vi "arm driver control.vi"(1 "Joystick Y":dbl) -> (0 "Setpoint":dbl)   [LabVIEW 2014]
uses:
  global variables/devrefs.vi
panel:
  # "Control the arm with PID setpoints instead of direct motor control"
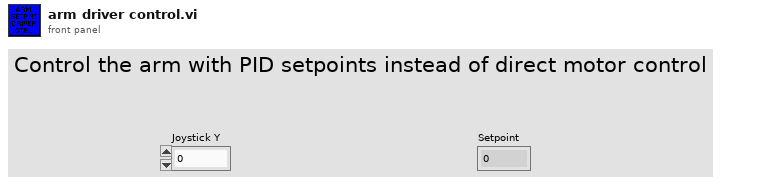
[diagram p1: front panel]
types:
  T1 = typedef "WPI_EncoderDevRef.ctl" = cluster{"DevStatus":errorcluster, "EncoderIndex":T2, "CounterIndex":T3, "DistancePerCount":dbl, "Decoding Type":T4}
  T2 = typedef "FPGA_EncoderIdx.ctl" = enum8{"Enc 0", "Enc 1", "Enc 2", "Enc 3", "Enc 4", "Enc 5", "Enc 6", "Enc 7", "Invalid"}
  T3 = typedef "FPGA_CounterCtrSystemIndex.ctl" = enum8{"Ctr 0", "Ctr 1", "Ctr 2", "Ctr 3", "Ctr 4", "Ctr 5", "Ctr 6", "Ctr 7", "Invalid"}
  T4 = typedef "WPI_EncoderType.ctl" = enum16{"1x", "2x", "4x"}
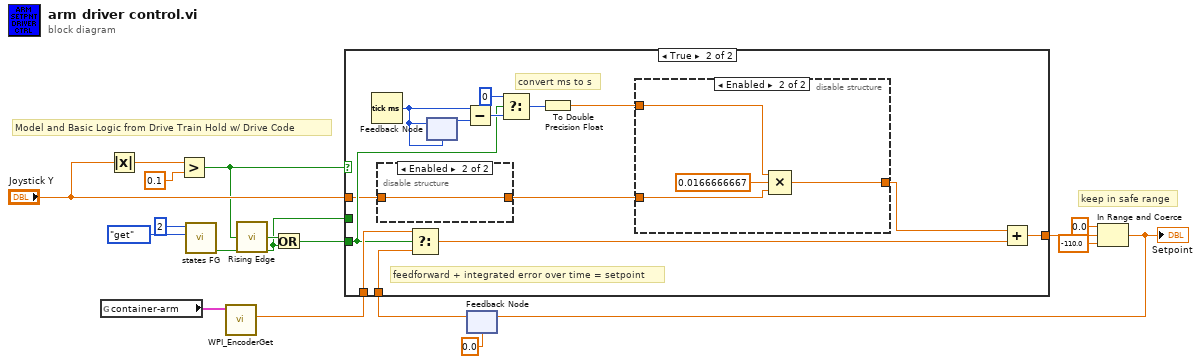
[diagram p0: block diagram]
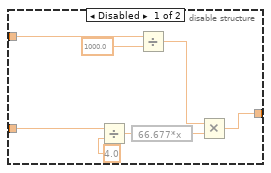
[diagram p4: hidden frame]
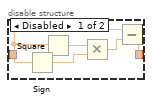
[diagram p5: hidden frame]
diagram:
  # "keep in safe range"
  # "Model and Basic Logic from Drive Train Hold w/ Drive Code"
  n1 = global read "devrefs.vi" "container-arm"() -> (w5:T1)
  n2 = Absolute Value(x="Joystick Y") -> (abs(x)=w16:dbl)
  n3 = Greater?(x=w16, y=0.1) -> (0:w10:bool)
  n4 = call "states FG.vi"("menu (get)"=enum16{"set", "get"}."get", "Loop ID"=2) -> ("first call?"=w6:bool)  [unwired: 6 in, 3 out]
  n5 = call <vilib>:"WPI_EncoderGet.vi"("EncoderDevRef"=w5) -> ("Distance"=w9:dbl)  [unwired: 5 in, 5 out]
  n6 = call "Rising Edge.vi"("Input"=w10) -> ("Rising Edge"=w12:bool)
  n7 = Or(x=w12, y=w6) -> (x .or. y?=w7:bool)
  n8 = feedback #1(0.0 ("upper limit")) -> (w8:dbl)
  n9 = case shown="True" w10 {
    tunnel: "Joystick Y" -> [_ w30]
    tunnel: w8 -> [w21 w35]
    tunnel: w7 -> [_ w31]
    tunnel: w9 -> [w20 w34]
    tunnel: [w19 w28] -> w4
    tunnel: w6 -> [w18 _]
    frame False {
      n10 = case shown="True" w18 {
        tunnel: w21 -> [w22 _]
        tunnel: w20 -> [_ w23]
        tunnel: [w22 w23] -> w19
        frame False {
          # "and get it there if it isn't there"
          # "hold arm at current commanded location"
        }
        frame True {
          # "hold arm at encoder location"
        }
      }
    }
    frame True {
      # "feedforward + integrated error over time = setpoint"
      # "convert ms to s"
      n11 = Tick Count (ms)() -> (millisecond timer value=w25:u32)
      n12 = disable-structure shown="Enabled" {
        disable-tunnel: w30 -> [w54 w55]
        disable-tunnel: [w53 w55] -> w27
        frame Disabled {
          n13 = Sign(1:w54) -> (0:w51:dbl)
          n14 = Square(x=w54) -> (x^2=w52:dbl)
          n15 = Multiply(x=w52, y=w51) -> (x*y=w50:dbl)
          n16 = Subtract(x=w54, y=w50) -> (x-y=w53:dbl)
        }
        frame Enabled {
        }
      }
      n17 = Select(t=w34, s=w31, f=w35) -> (s? t:f=w29:dbl)
      n18 = feedback #2(w25) -> (w26:u32)
      n19 = feedback-in #2(w25) -> ()
      n20 = Subtract(x=w25, y=w26) -> (x-y=w36:u32)
      n21 = Select(t=u32 0, s=w31, f=w36) -> (s? t:f=w32:u32)
      n22 = To Double Precision Float(number=w32) -> (double precision float=w33:dbl)
      n23 = disable-structure shown="Enabled" {
        disable-tunnel: w33 -> [w45 w49]
        disable-tunnel: w27 -> [w41 w48]
        disable-tunnel: [w38 w46] -> w24
        frame Disabled {
          n24 = Divide(x=w41, y=4.0) -> (x/y=w40:dbl)
          n25 = expression code="66.677*x"(w40) -> (w39:dbl)
          n26 = Divide(x=w45, y=1000.0) -> (x/y=w43:dbl)
          n27 = Multiply(x=w43, y=w39) -> (x*y=w38:dbl)
        }
        frame Enabled {
          n28 = Compound Arithmetic op=MULTIPLY(w49, 0.0166666667 ("value"), w48) -> (w46:dbl)
        }
      }
      n29 = Add(x=w24, y=w29) -> (x+y=w28:dbl)
    }
  }
  n30 = In Range and Coerce(upper limit=0.0, x=w4, lower limit=-110.0) -> (coerced(x)=w3:dbl)  [unwired: 1 out]
  "Setpoint" <- w3
  n31 = feedback-in #1(w3) -> ()
